vi "LVProjectShortcut_Item_OnDblClick.vi"(11 "Object":T1) -> ()   [LabVIEW 2017, in "LVProject Shortcut.lvlib"]
uses:
  <resource>/Framework/Providers/API/ItemRef.ctl
  LVProject Shortcut.lvlib
panel:
  out "error out":errorcluster
  in  "error in":errorcluster
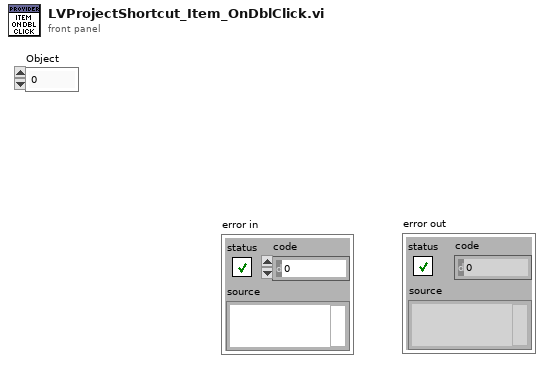
[diagram p1: front panel]
types:
  T1 = typedef "ItemRef.ctl" = u64
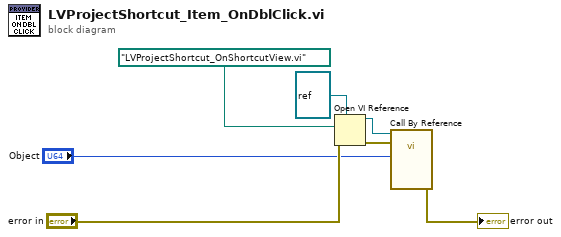
[diagram p0: block diagram]
diagram:
  n1 = Open VI Reference(type specifier VI Refnum (for type only)=refnum<vi> refnum, vi path=path "LVProjectShortcut_OnShortcutView.vi", error in (no error)="error in") -> (vi reference=w2:refnum<vi>, error out=w7:errorcluster)  [unwired: 3 in]
  n2 = call-by-ref "?"(reference=w2, error in=w7, "Object"="Object") -> (error out=→"error out":errorcluster)  [unwired: 10 in, 2 out]
